vi "_2D array to HTML.vi"(7 "Table (2D Array)":string[][](table)=[["[Step 1]"], ["[Step 2]"], ["[Step 3]"], ["[Step 4]"]]) -> (8 "HTML Code":string)   [LabVIEW 2012]
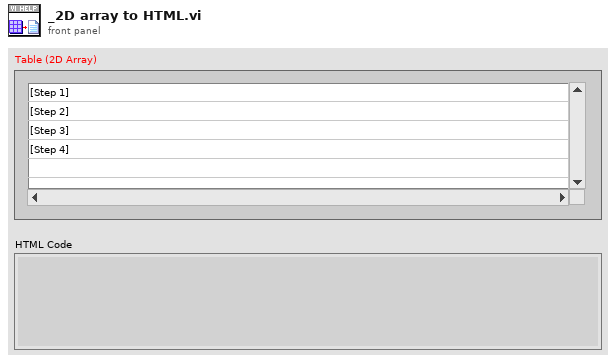
[diagram p1: front panel]
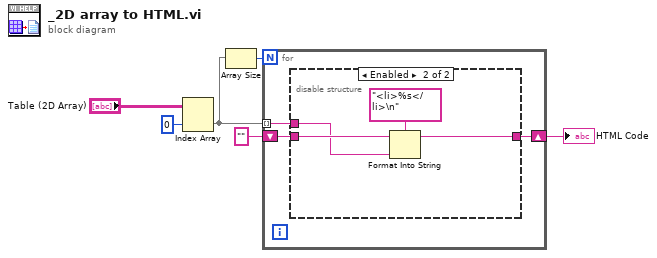
[diagram p0: block diagram]
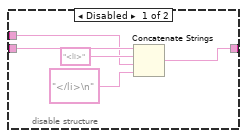
[diagram p2: hidden frame]
diagram:
  n1 = Index Array(array="Table (2D Array)", index (col)=0 ("index (row)")) -> (element=w4:string[])  [unwired: 1 in]
  n2 = Array Size(array=w4) -> (size(s)=w5:i32)
  n3 = for {
    N: w5 -> [_]
    tunnel: w4 -> [w8] mode=indexing
    shift-right: [w7] -> w2
    shift-left: "" -> [w9]
    n4 = disable-structure shown="Enabled" {
      disable-tunnel: w9 -> [w14 w17]
      disable-tunnel: w8 -> [w12 w16]
      disable-tunnel: [w10 w15] -> w7
      frame Disabled {
        n5 = Concatenate Strings(w14, "<li>" ("string"), w12, "</li>\n" ("string")) -> (w10:string)
      }
      frame Enabled {
        n6 = Format Into String(format string="<li>%s</li>\n", initial string=w17, w16) -> (resulting string=w15:string)  [unwired: 1 in, 1 out]
      }
    }
  }
  "HTML Code" <- w2
